vi "Number to String Bar Graph.vi"(0 "Scale Max":dbl, 5 "Numeric":dbl, 7 "Scale Min":dbl) -> (6 "element":string)   [LabVIEW 2019, in "Instrument.Lockin.lvclass"]
uses:
  Instrument.Lockin.lvclass
  <vilib>/Analysis/1siggen.llb/Ramp Pattern by Samples.vi
  <vilib>/Analysis/NI_AALBase.lvlib
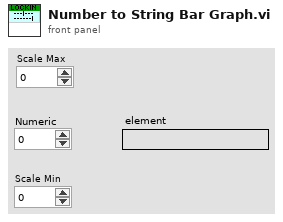
[diagram p1: front panel]
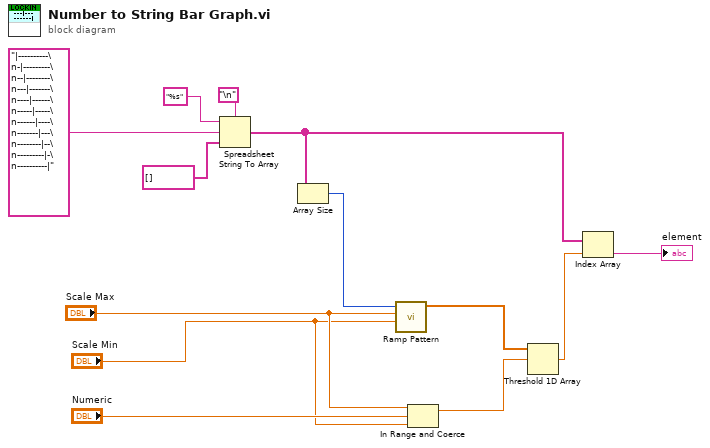
[diagram p0: block diagram]
diagram:
  n1 = Spreadsheet String To Array(delimiter (Tab)="\n", format string="%s", spreadsheet string="|----------\n-|---------\n--|--------\n---|-------\n----|------\n-----|-----\n------|----\n-------|---\n--------|--\n---------|-\n----------|" ("spinner 4"), array type (2D Dbl)=string[] []) -> (array=w2:string[])
  n2 = Array Size(array=w2) -> (size(s)=w9:i32)
  n3 = call-poly <vilib>:"Ramp Pattern.vi"("start"="Scale Min", "end"="Scale Max", "samples"=w9) -> ("Ramp Pattern"=w8:dbl[])  [unwired: 7 in, 1 out]
  n4 = In Range and Coerce(upper limit="Scale Max", x="Numeric", lower limit="Scale Min") -> (coerced(x)=w4:dbl)  [unwired: 1 out]
  n5 = Threshold 1D Array(2:w4, 3:w8) -> (0:w3:dbl)  [unwired: 1 in]
  n6 = Index Array(array=w2, index=w3) -> (element=→"element":string)
